vi "Open VI Panel.vi"(8 "error in":errorcluster, 11 "VI":refnum<vi>) -> (0 "error out":errorcluster)   [LabVIEW 2026, in "CML UI.lvlib"]
doc: "Open and activate the panel of the specified VI.\n_____\nBased on DQMH Project Template 4.0.0.47.\n_____\nBased on DQMH Dev Tools: Project Template 7.1.2.1547."
uses:
  CML UI.lvlib
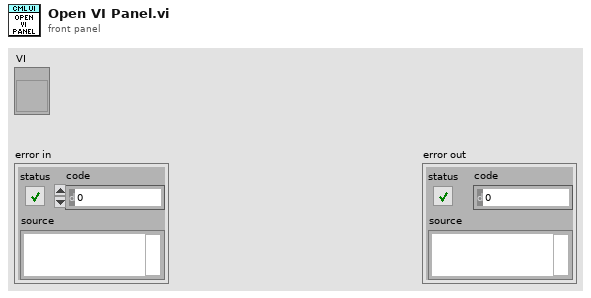
[diagram p1: front panel]
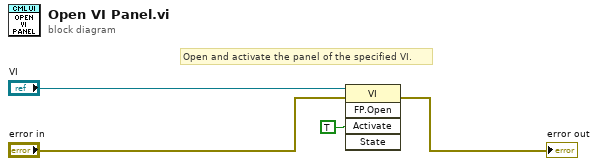
[diagram p0: block diagram]
diagram:
  # "Open and activate the panel of the specified VI."
  n1 = invoke on="Invoke Node" class="VI" method="FP.Open"(reference="VI", error in="error in", "Activate"=TRUE ("Activate?")) -> (error out=→"error out":errorcluster)  [unwired: 2 in, 4 out]
